vi "SVT Peak Level (N Ch).vi"(6 "restart averaging (F)":bool, 8 "error in (no error)":errorcluster, 11 "scaled signals [EU]":waveform(dbl)[](array[waveform])) -> (0 "error out":errorcluster, 2 "unit labels":string[](array[string]), 3 "peak levels [EU]":dbl[](array[numeric]) format="%.2f")   [LabVIEW 2017]
doc: "Computes the peak level of <B>scaled signal [EU]</B> or <B>even angle signal [EU]</B>. You can use this polymorphic VI to compute the peak level for a single channel or for N channels, or for a single channel or N channels of angular resampled data. The data type you wire to the <B>scaled signal [EU]</B> or <B>even angle signal [EU]</B> input determines the polymorphic instance to use."
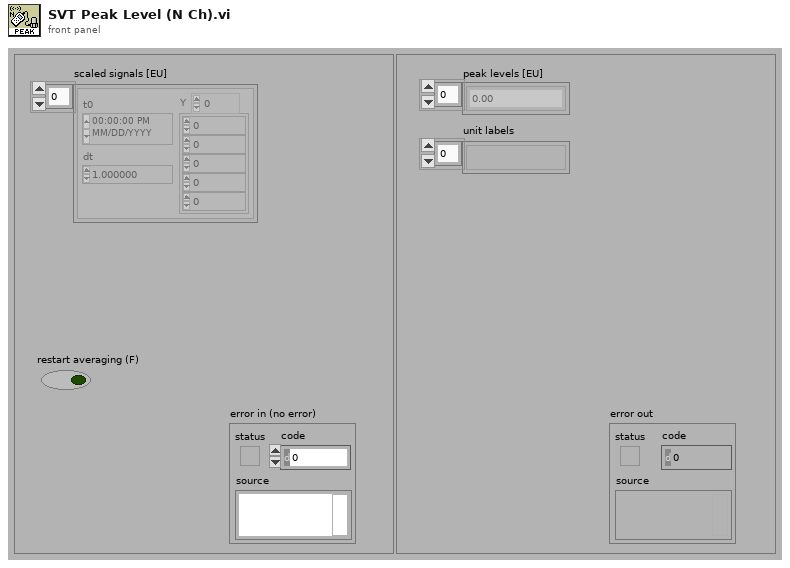
[diagram p1: front panel]
types:
  T1 = enum16{"RMS", "Running RMS", "Exp avg  ", "Dec exp avg ", "Peak", "Crest"}
  T2 = enum16{"Reset filter", "Restart averaging", "Continue processing"}
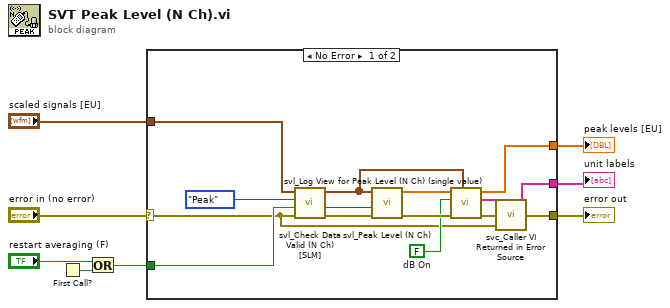
[diagram p0: block diagram]
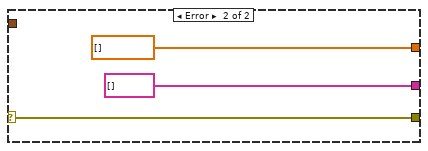
[diagram p2: hidden frame]
diagram:
  n1 = First Call?() -> (First Call?: T/F=w4:bool)
  n2 = Or(x="restart averaging (F)", y=w4) -> (x .or. y?=w2:bool)
  n3 = case shown="No Error" "error in (no error)" {
    selector: "error in (no error)" -> [w9 w25]
    tunnel: [w17 w25] -> w8
    tunnel: [w21 string[] [] ("unit label [ ]")] -> w7
    tunnel: [w20 dbl[] [] ("energy levels [EU^2 rms]")] -> w6
    tunnel: "scaled signals [EU]" -> [w11 _]
    tunnel: w2 -> [w15 _]
    frame No Error {
      w13 = FALSE  # dB On
      n4 = call <vilib>:"svl_Check Data Valid (N Ch) [SLM].vi"("error in (no error)"=w9, "restart averaging (F)"=w15, "level analysis"=T1."Peak" ("Level Analysis"), "scaled signals [EU]"=w11) -> ("error out"=w16:errorcluster, "processing state"=w14:T2, "dup scaled signals [EU]"=w10:waveform(dbl)[])  [unwired: 5 in]
      n5 = call <vilib>:"svl_Peak Level (N Ch).vi"("error in (no error)"=w16, "processing state"=w14, "scaled signals [EU]"=w10) -> ("error out"=w18:errorcluster, "peak levels"=w19:dbl[])  [unwired: 7 in]
      n6 = call <vilib>:"svl_Log View for Peak Level (N Ch) (single value).vi"("scaled signals [EU]"=w10, "error in (no error)"=w18, "dB On (T)"=w13, "peak levels [EU]"=w19) -> ("error out"=w22:errorcluster, "unit label [ ]"=w21:string[], "peak levels [EU]"=w20:dbl[])  [unwired: 5 in]
      n7 = call <vilib>:"svc_Caller VI Returned in Error Source.vi"("warning input to caller"=w9, "error in (no error)"=w22) -> ("error out"=w17:errorcluster)  [unwired: 3 in]
    }
    frame Error {
    }
  }
  "peak levels [EU]" <- w6
  "unit labels" <- w7
  "error out" <- w8
